vi "peis.vi"(5 "Draw":T2(ring), 6 "DLLPath":path, 7 "Channel":u8(ring) items=["1", "2", "3", "4", "5", "6", "7", "8", "9", "10", "11", "12", "13", "14", "15", "16"], 8 "error in (no error)":errorcluster, 9 "PEIS Parameters":T3={"Step_number"=0, "Initial_Voltage_step"=0.0, "vs_initial"=TRUE, "Final_Voltage_step"=1.0, "vs_final"=FALSE, "Duration_step"=1.0, "Record_every_dI"=0.1, "Record_every_dT"=0.1, "Initial_frequency"=100000.0, "sweep"=FALSE, "Final_frequency"=1.0, "Frequency_number"=51, "Amplitude_Voltage"=0.01, "Wait_for_steady"=2.0, "Average_N_times"=1, "Correction"=TRUE, "I_Range"=12, "Bandwidth"=5, "em"=1, "ce"=0} {"ce" items=["Standard", "CE to ground"]; "Initial_Voltage_step" min=-10 max=10 format="%.5f"; "Step_number" min=0 step=1; "I_Range" items=["1pA", "1nA", "10nA", "100nA", "1µA", "10µA", "100µA", "1mA", "10mA", "100mA", "1A", "Booster", "Auto"]; "Wait_for_steady" min=0 format="%.2f"; "Record_every_dT" min=0 format="%.2e"; "Record_every_dI" min=0 format="%.2e"; "Duration_step" min=0 format="%.5f"; "Final_Voltage_step" min=-10 max=10 format="%.5f"; "Bandwidth" items=["1"=1, "2"=2, "3"=3, "4"=4, "5"=5, "6"=6, "7"=7, "8"=8, "9"=9]; "Average_N_times" min=1 max=1000 step=1; "Amplitude_Voltage" min=0.0005 max=0.5 format="%.2e"; "Final_frequency" min=1e-05 max=1000000 format="%.2e"; "Frequency_number" min=1 max=10000; "Initial_frequency" min=1e-05 max=1000000 format="%.2e"}, 11 "IP adress":string="192.109.209.229") -> (0 "error out":errorcluster, 2 "Exit 2":bool=TRUE, 3 "XY Graph":cluster{"Data p1":sgl[], "Data p1":dbl[]}[](graph), 4 "Data":T1)   [LabVIEW 2022 SP3]
doc: "The Staircase Potentio Electrochemical Impedance Spectroscopy (SPEIS) technique is designed to perform successive impedance measurements (on a whole frequency range) during a potential sweep. \nThis technique consists in a staircase potential sweep (potential limits and number of steps defined by the user). An impedance measurement (with an adjustable number of frequencies) is performed on each potential step.\n\nIn general, in this VI, the first thing to do is to start by establishing the connection with the instrument defined by its IP adress, then load the firmware in the channel selected, get the information on the plugged channels, load protocol on a channel, start/stop the protocol, retreive data and draw the graph.\nThis technique is applied just for channels with impedance capabilities (Zboard)."
uses:
  Library/EClib Functions/PEISParameters.ctl
  Library/EClib Functions/Parameters.ctl
  Library/EClib Functions/EClib functions.lvlib
panel:
  in  "Display Parameters?":bool caption="Display Parameters"
  out "DllPath":path caption="DLL Path"
  out "LibVersion":string caption="DLL Version"
  out "Number of points":i32=52
  out "Data p0":sgl[][](array[numeric])=[[0.100008, 0.099745475, 1.9343544e-05], [0.200016, 0.09966919, 1.936642e-05], [0.300024, 0.10005063, 1.9374045e-05], [0.400032, 0.10005063, 1.9358795e-05], [0.50004, 0.09997434, 1.9358795e-05], [0.600048, 0.09982177, 1.938167e-05], [0.700056, 0.099516615, 1.9358795e-05], [0.800064, 0.099898055, 1.9374045e-05], [0.90007204, 0.099516615, 1.936642e-05]]
  out "Data p1":sgl[][](array[numeric])=[[99999.99, 0.009897927, 1.5485124e-05, -0.23932889, 0.09957624, 2.0601647e-05, 0.0, 0.017584162, 1.5528842e-05, -0.13801742, -0.10928005, -2.0601661e-05, 0.0, 1.89, 7.0], [79789.055, 0.009909321, 1.4999416e-05, -0.28277892, 0.09956935, 2.0610883e-05, 0.0, 0.017358849, 1.5026583e-05, -0.16497254, -0.10927754, -2.0610896e-05, 0.0, 2.319, 7.0], [63671.867, 0.00993305, 1.4371862e-05, -0.3338619, 0.099571265, 2.0617736e-05, 0.0, 0.01701651, 1.4388475e-05, -0.19887781, -0.10927467, -2.0617748e-05, 0.0, 2.748, 7.0], [50804.684, 0.009895762, 1.349999e-05, -0.38682938, 0.099595726, 2.0621628e-05, 0.0, 0.016509676, 1.3509973e-05, -0.23511207, -0.10929042, -2.0621641e-05, 0.0, 3.177, 7.0], [40539.06, 0.009924297, 1.2531375e-05, -0.43154812, 0.09956674, 2.0623062e-05, 0.0, 0.01605967, 1.2537333e-05, -0.27001935, -0.1092824, -2.0623074e-05, 0.0, 3.606, 7.0], [32343.752, 0.009929493, 1.1422184e-05, -0.4605673, 0.099575475, 2.0627644e-05, 0.0, 0.015497766, 1.1425662e-05, -0.29694676, -0.10927959, -2.0627656e-05, 0.0, 4.035, 7.0], [25812.496, 0.009931898, 1.0332502e-05, -0.47349262, 0.09957423, 2.0616248e-05, 0.0, 0.014982226, 1.0334525e-05, -0.31350675, -0.10928383, -2.0616259e-05, 0.0, 4.4639997, 7.0], [20593.748, 0.009683827, 9.104932e-06, -0.46709442, 0.09957324, 2.0613099e-05, 0.0, 0.014134236, 9.106069e-06, -0.3174526, -0.10928545, -2.0613114e-05, 0.0, 4.75, 7.0], [16429.69, 0.00984061, 8.381006e-06, -0.4425385, 0.0995779, 2.0614962e-05, 0.0, 0.013980997, 8.381673e-06, -0.30736777, -0.10928426, -2.0614974e-05, 0.0, 5.036, 7.0], [13109.373, 0.009880392, 7.759602e-06, -0.4042132, 0.09956233, 2.0629059e-05, 0.0, 0.013766184, 7.759997e-06, -0.28469434, -0.10927877, -2.0629072e-05, 0.0, 5.322, 7.0], [10460.936, 0.009915135, 7.290463e-06, -0.35881066, 0.099576354, 2.062228e-05, 0.0, 0.013552605, 7.2907023e-06, -0.25464892, -0.10927802, -2.0622294e-05, 0.0, 5.608, 7.0], [8351.5625, 0.009958473, 6.968417e-06, -0.30687237, 0.09957134, 2.0619169e-05, 0.0, 0.013452288, 6.968562e-06, -0.21966934, -0.10928822, -2.0619183e-05, 0.0, 5.894, 7.0], [6660.1553, 0.009773157, 6.585265e-06, -0.26302314, 0.09957721, 2.0628519e-05, 0.0, 0.013077308, 6.5853465e-06, -0.18975565, -0.109301746, -2.0628531e-05, 0.0, 6.0620003, 7.0], [5313.953, 0.009875495, 6.4977903e-06, -0.21722555, 0.09959636, 2.061105e-05, 0.0, 0.013129692, 6.497844e-06, -0.15612268, -0.10930546, -2.0611064e-05, 0.0, 6.269, 7.0], [4241.786, 0.009916322, 6.4091464e-06, -0.17841792, 0.09959986, 2.0643229e-05, 0.0, 0.013149473, 6.4091746e-06, -0.12683374, -0.109303646, -2.0643243e-05, 0.0, 6.4830003, 7.0], [3385.4163, 0.009962957, 6.371731e-06, -0.15283132, 0.09959816, 2.0641255e-05, 0.0, 0.013166811, 6.371748e-06, -0.11219756, -0.10930573, -2.0641268e-05, 0.0, 6.697, 7.0], [2699.3184, 0.009985389, 6.3324687e-06, -0.12883663, 0.099599674, 2.0642745e-05, 0.0, 0.013169419, 6.3324833e-06, -0.09362733, -0.10931173, -2.0642758e-05, 0.0, 6.9110003, 7.0], [2153.4448, 0.009996085, 6.3133293e-06, -0.11305499, 0.09959159, 2.0643656e-05, 0.0, 0.013185124, 6.313335e-06, -0.08275235, -0.109307505, -2.064367e-05, 0.0, 7.125, 7.0], [1717.748, 0.010014333, 6.2567524e-06, -0.10080016, 0.09959457, 2.0655203e-05, 0.0, 0.013182044, 6.256763e-06, -0.07431483, -0.10931141, -2.0655216e-05, 0.0, 7.34, 7.0], [1372.1951, 0.010016238, 6.2877625e-06, -0.09321749, 0.09959682, 2.064688e-05, 0.0, 0.013175669, 6.2877634e-06, -0.06877315, -0.10931128, -2.0646892e-05, 0.0, 7.5550003, 7.0], [1096.7545, 0.010012516, 6.286433e-06, -0.08541584, 0.09960139, 2.0640491e-05, 0.0, 0.013178928, 6.2864306e-06, -0.062073976, -0.10930484, -2.0640506e-05, 0.0, 7.77, 7.0], [871.93097, 0.010010969, 6.268487e-06, -0.08781743, 0.09959833, 2.0634905e-05, 0.0, 0.013172707, 6.2684835e-06, -0.06440747, -0.109307244, -2.0634918e-05, 0.0, 7.987, 7.0], [696.1138, 0.01003125, 6.2508416e-06, -0.093888, 0.09959319, 2.0650714e-05, 0.0, 0.013164024, 6.2508466e-06, -0.069969416, -0.10931639, -2.0650728e-05, 0.0, 8.203, 7.0], [555.8894, 0.010025321, 6.2520185e-06, -0.10746312, 0.099596396, 2.063822e-05, 0.0, 0.01315077, 6.2520166e-06, -0.08037281, -0.109306626, -2.0638234e-05, 0.0, 8.42, 7.0], [443.43906, 0.010033136, 6.209101e-06, -0.12175393, 0.0995993, 2.0631758e-05, 0.0, 0.01312816, 6.2091035e-06, -0.091670275, -0.109299496, -2.063177e-05, 0.0, 8.639, 7.0], [353.75473, 0.01003465, 6.1840165e-06, -0.14335668, 0.09959073, 2.0645593e-05, 0.0, 0.013097799, 6.1840187e-06, -0.10758209, -0.10931424, -2.0645608e-05, 0.0, 8.859, 7.0], [281.8943, 0.010030967, 6.109471e-06, -0.17281115, 0.09959446, 2.0650212e-05, 0.0, 0.013065848, 6.109473e-06, -0.129511, -0.10930905, -2.0650225e-05, 0.0, 9.0789995, 7.0], [225.3606, 0.010023677, 6.0119432e-06, -0.20512176, 0.09959748, 2.064375e-05, 0.0, 0.013001974, 6.0119396e-06, -0.15545309, -0.1093129, -2.0643763e-05, 0.0, 9.301, 7.0], [180.28844, 0.010028235, 5.913567e-06, -0.25207758, 0.0995884, 2.0643136e-05, 0.0, 0.012923154, 5.913563e-06, -0.19031943, -0.1093126, -2.0643149e-05, 0.0, 9.526, 7.0], [143.75787, 0.010025335, 5.723294e-06, -0.2980666, 0.09959362, 2.0638052e-05, 0.0, 0.012791262, 5.7232987e-06, -0.22673774, -0.109312676, -2.0638066e-05, 0.0, 9.755, 7.0], [114.59661, 0.0100282775, 5.478785e-06, -0.36026663, 0.09959826, 2.0642558e-05, 0.0, 0.012615283, 5.4787893e-06, -0.27884817, -0.109307505, -2.0642572e-05, 0.0, 9.987, 7.0], [91.552734, 0.010020258, 5.1631105e-06, -0.41180015, 0.09958356, 2.0632298e-05, 0.0, 0.012400166, 5.1631077e-06, -0.32256132, -0.10930771, -2.0632311e-05, 0.0, 10.219, 7.0], [72.87778, 0.010045694, 4.7920767e-06, -0.47027957, 0.0995903, 1.9318108e-05, 0.0, 0.012195916, 4.7920753e-06, -0.37585485, -0.10930665, -1.931812e-05, 0.0, 10.735, 6.0], [58.30223, 0.010017018, 4.3459513e-06, -0.5196618, 0.09958969, 1.931711e-05, 0.0, 0.011869716, 4.345951e-06, -0.41790736, -0.109305374, -1.9317124e-05, 0.0, 10.989, 6.0], [46.50297, 0.010043655, 3.8964367e-06, -0.5461425, 0.09958527, 1.9321726e-05, 0.0, 0.011661541, 3.8964395e-06, -0.45622373, -0.10929812, -1.9321737e-05, 0.0, 11.24, 6.0], [36.95101, 0.0100237075, 3.4589034e-06, -0.55786407, 0.09959118, 1.9322812e-05, 0.0, 0.011445447, 3.4589052e-06, -0.47548974, -0.1093029, -1.9322824e-05, 0.0, 11.498, 6.0], [29.592804, 0.010024518, 3.0782626e-06, -0.5442606, 0.099590674, 1.9320825e-05, 0.0, 0.011281099, 3.0782635e-06, -0.4723431, -0.10930497, -1.9320838e-05, 0.0, 11.782001, 6.0], [23.588463, 0.010025413, 2.7635026e-06, -0.50970626, 0.09959939, 1.931987e-05, 0.0, 0.011168829, 2.7635024e-06, -0.45203626, -0.10930516, -1.9319881e-05, 0.0, 12.092, 6.0], [18.780045, 0.010028319, 2.5114025e-06, -0.46162716, 0.0995976, 1.9318664e-05, 0.0, 0.01109292, 2.5114036e-06, -0.4128492, -0.109315775, -1.9318675e-05, 0.0, 12.425, 6.0], [15.024037, 0.010029642, 2.331001e-06, -0.4064955, 0.099582985, 1.9321948e-05, 0.0, 0.01104459, 2.3310024e-06, -0.36793888, -0.10930361, -1.9321958e-05, 0.0, 12.772, 6.0], [11.982363, 0.010013976, 2.1986236e-06, -0.3445742, 0.0995901, 1.9318428e-05, 0.0, 0.01101896, 2.198625e-06, -0.31417423, -0.10929007, -1.931844e-05, 0.0, 13.119, 6.0], [9.574144, 0.010021789, 2.1110484e-06, -0.29042864, 0.09959056, 1.931938e-05, 0.0, 0.011009957, 2.1110482e-06, -0.26570365, -0.10930588, -1.9319392e-05, 0.0, 13.55, 6.0], [7.6293964, 0.010015764, 2.047544e-06, -0.2358973, 0.09959619, 1.9324216e-05, 0.0, 0.010986972, 2.0475438e-06, -0.21676749, -0.10930043, -1.9324229e-05, 0.0, 14.088, 6.0], [6.084501, 0.010008753, 2.0095065e-06, -0.19609833, 0.09960107, 1.9321422e-05, 0.0, 0.010978085, 2.0095063e-06, -0.17923641, -0.10930903, -1.9321435e-05, 0.0, 14.758, 6.0], [4.858519, 0.0100127505, 1.9834858e-06, -0.15383446, 0.099605374, 1.9325236e-05, 0.0, 0.01099137, 1.983485e-06, -0.14275539, -0.10930968, -1.9325249e-05, 0.0, 15.594, 6.0], [3.8752477, 0.010018873, 1.964741e-06, -0.12660927, 0.09960577, 1.9319072e-05, 0.0, 0.01098087, 1.9647398e-06, -0.11773729, -0.10930894, -1.9319084e-05, 0.0, 16.639, 6.0], [3.1001983, 0.01002199, 1.954336e-06, -0.101673305, 0.09960291, 1.9318823e-05, 0.0, 0.010977447, 1.9543347e-06, -0.09406805, -0.10931086, -1.9318833e-05, 0.0, 17.943, 6.0], [2.4660668, 0.010017678, 1.9471984e-06, -0.08063111, 0.09960053, 1.9318097e-05, 0.0, 0.010982101, 1.9471975e-06, -0.07494378, -0.10931104, -1.9318108e-05, 0.0, 19.579, 6.0], [1.9649143, 0.01001538, 1.9460967e-06, -0.064157724, 0.09960199, 1.9316354e-05, 0.0, 0.010980325, 1.946096e-06, -0.06017399, -0.1093061, -1.9316365e-05, 0.0, 21.627, 6.0], [1.5725644, 0.010012327, 1.941652e-06, -0.051375534, 0.09960348, 1.9317453e-05, 0.0, 0.010977772, 1.9416514e-06, -0.04843211, -0.10930792, -1.9317464e-05, 0.0, 24.183, 6.0], [1.2520034, 0.010019626, 1.939335e-06, -0.041469768, 0.09961237, 1.9318904e-05, 0.0, 0.010981496, 1.9393347e-06, -0.038478374, -0.109313786, -1.9318915e-05, 0.0, 27.391, 6.0], [1.0016024, 0.010014649, 1.938777e-06, -0.033258826, 0.09960662, 1.931856e-05, 0.0, 0.010977961, 1.9387764e-06, -0.031450033, -0.109310396, -1.9318572e-05, 0.0, 31.398, 6.0]]
  in  "stop":bool
  in  "Exit":bool
  in  "Start":bool
  # "Instructions:\nBefore running the VI you must type a valid IP adress that corresponds to the instrument.Then press the Run button to execute this VI.\nWhile this VI is running, choose the available channel, enter the SPEIS parameters or keep the default\n values, then press the start button to begin the experience. \nChoose the waveform to draw : Nyquist, modZ, theta...\nPress the stop button to end experience and the exit button to stop the VI execution."
  # "Set E (V)  vs. previous"
  # "Before EIS  stay for ts (s)"
  # "and record every dI (A)"
  # "or every dt (s)"
  # "Start EIS from  Fi (Hz)"
  # "sweep linear/logarithmic"
  # "to Ff (Hz)"
  # "for Nf frequencies"
  # "with the amplitude (V)"
  # "wait for Pw"
  # "average Na times"
  # "drift correction"
  # "with I Range"
  # "and bandwidth"
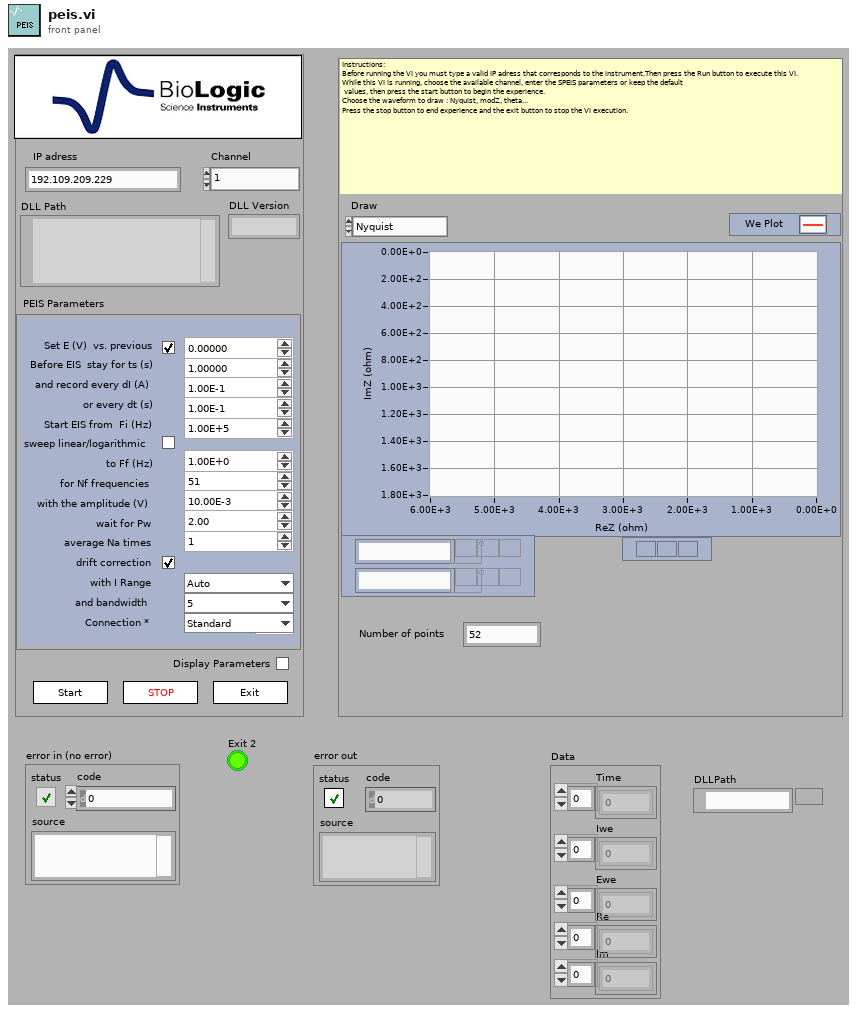
[diagram p1: front panel]
types:
  T1 = cluster{"Time":sgl[], "Iwe":sgl[], "Ewe":sgl[], "Re":sgl[], "Im":sgl[]}
  T2 = enum16{"Nyquist", "modZ", "theta", "modE", "modI", "Edc", "Idc", "E range", "I range", "f(t)", "Test"}
  T3 = typedef "EClib functions.lvlib/PEISParameters.ctl" = cluster{"Step_number":i32, "Initial_Voltage_step":sgl, "vs_initial":bool, "Final_Voltage_step":sgl, "vs_final":bool, "Duration_step":sgl, "Record_every_dI":sgl, "Record_every_dT":sgl, "Initial_frequency":sgl, "sweep":bool, "Final_frequency":sgl, "Frequency_number":i32, "Amplitude_Voltage":sgl, "Wait_for_steady":sgl, "Average_N_times":i32, "Correction":bool, "I_Range":u16, "Bandwidth":u16, "em":u16, "ce":u16}
  T4 = cluster{"LibVersion":string, "StringLength":u32, "DllPath":path}
  T5 = cluster{"Channel":i32, "BoardVersion":i32, "BoardSerialCode":i32, "FirmwareCode":i32, "FirmwareVersion":i32, "XilinxVersion":i32, "AmpCode":i32, "NbAmp":i32, "LcBoard":i32, "Zboard":i32, "MuxBoard":i32, "GPRAboard":i32, "MemSize":i32, "MemFilled":i32, "state":i32, "MaxIRange":i32, "MinIRange":i32, "MaxBandwidth":i32, "NbOfTechniques":i32}
  T6 = typedef "EClib functions.lvlib/Parameters.ctl" = enum16{"CA", "CASG", "CP", "GEIS", "ISCAN", "OCV", "PEIS", "SCCX", "SGEIS", "SPEIS", "VSCAN", "MP"}
  T7 = typedef "EClib functions.lvlib/TechniqueParameters.ctl" = cluster{"String Label":string, "Type":i32, "Valeur":i32, "Index":i32}
  T8 = cluster{"string before end tag":string, i32, i32, i32}[]
  T9 = cluster{"IRQskipped":i32, "NbRaws":i32, "NbCols":i32, "Technique Index":i32, "TechniqueID":i32, "PrcessIndex":i32, "loop":i32, "StartTime":dbl, "MuxPad":i32}
  T10 = cluster{"State":i32, "MemFilled":i32, "TimeBase":sgl, " Ewe":sgl, " EweRangeMin":sgl, " EweRangeMax":sgl, "Ece":sgl, "EceRangeMin":sgl, "EceRangeMax":sgl, "Eoverflow":i32, "I":sgl, "IRange":i32, "Ioverflow":i32, "ElapsedTime":sgl, "Freq":sgl, "Rcomp":sgl, "Saturation":sgl, "OptErr":i32, "OptPos":i32}
  T11 = cluster{"Data p0":sgl[], "Data p0":sgl[], "Data p0":sgl[], sgl[], sgl[]}
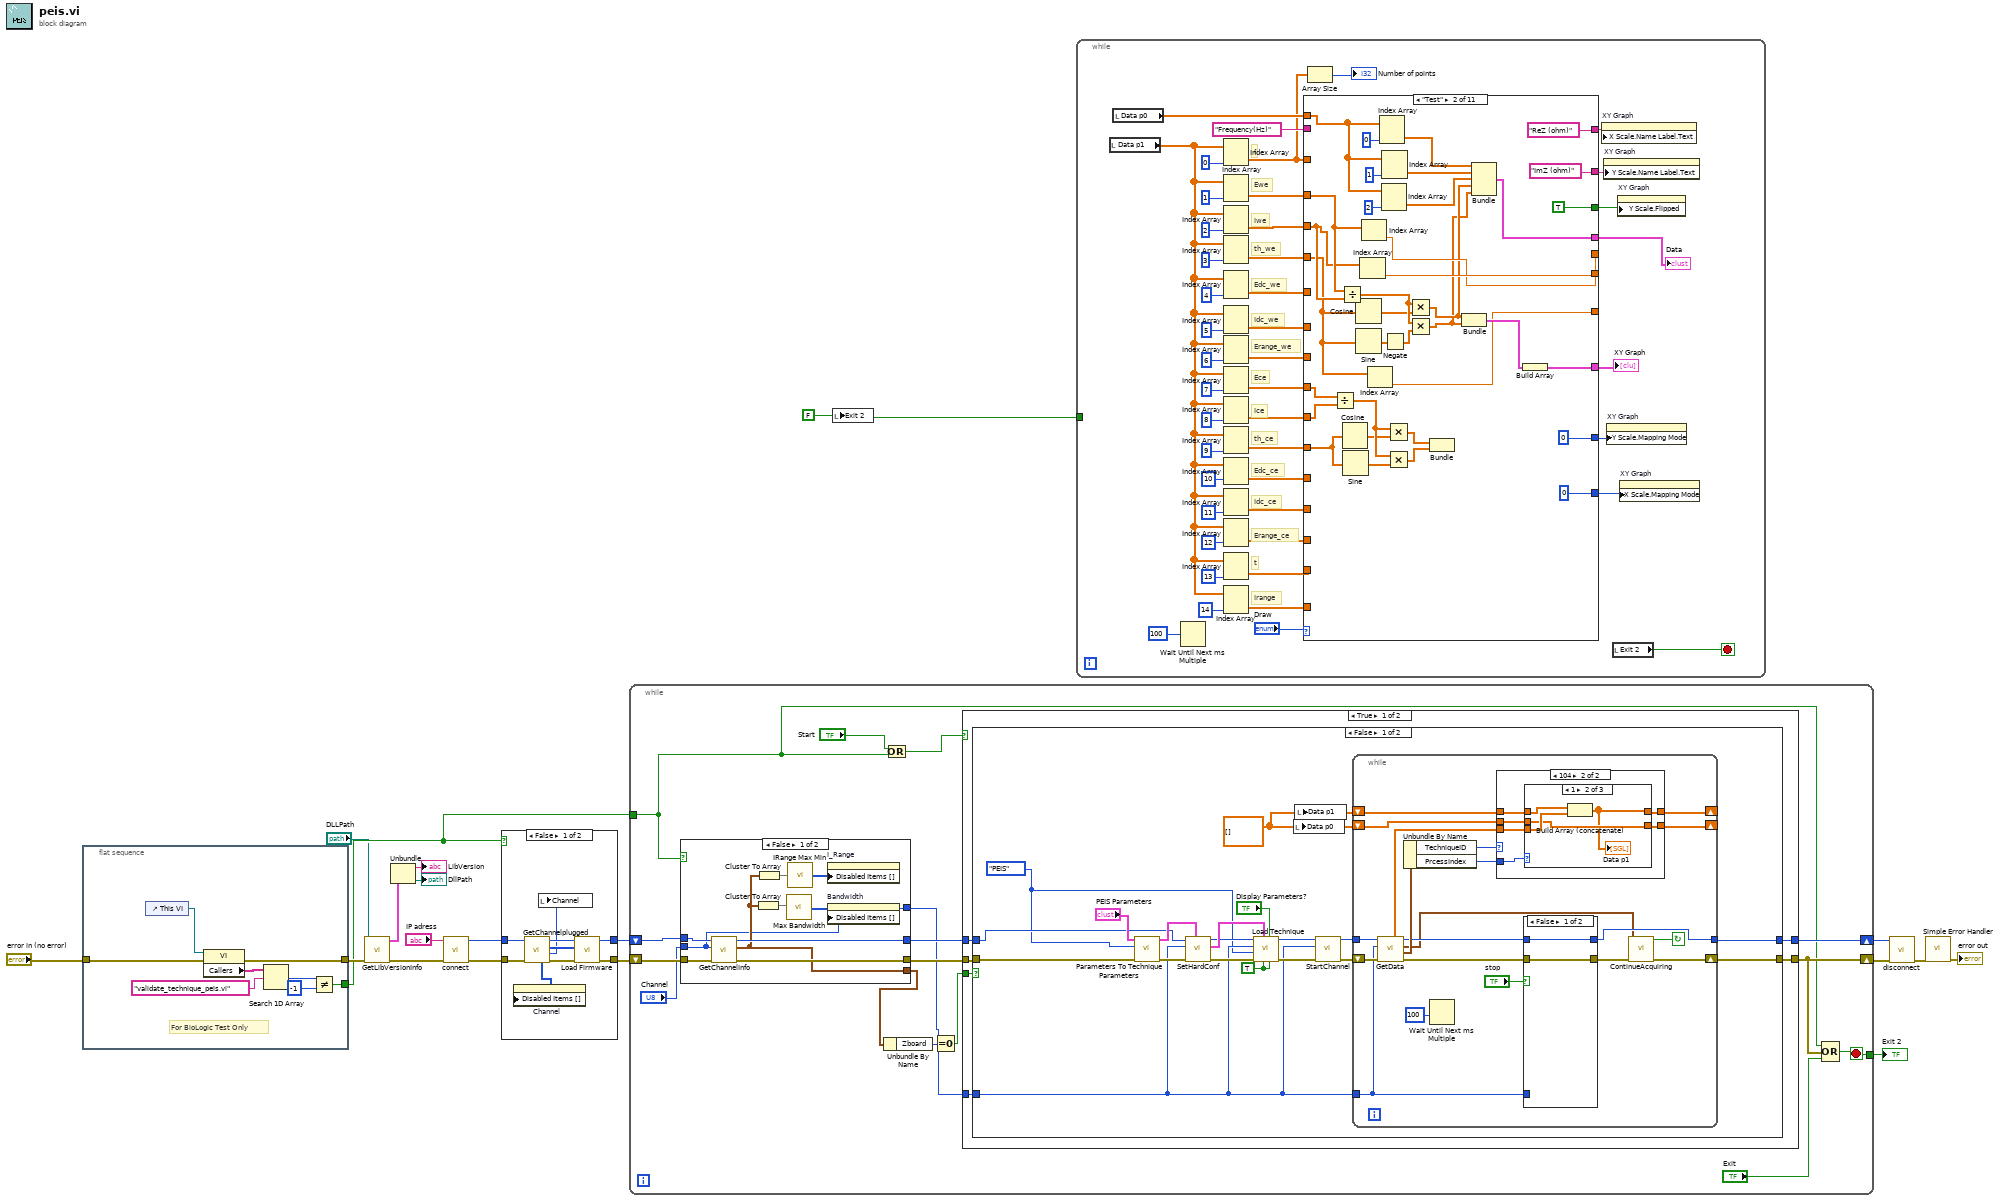
[diagram p0: block diagram]
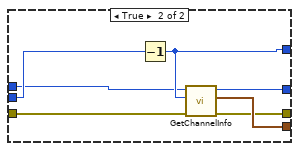
[diagram p3: hidden frame]
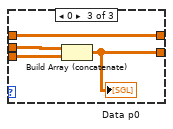
[diagram p6: hidden frame]
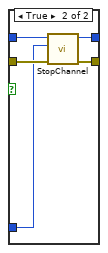
[diagram p7: hidden frame]
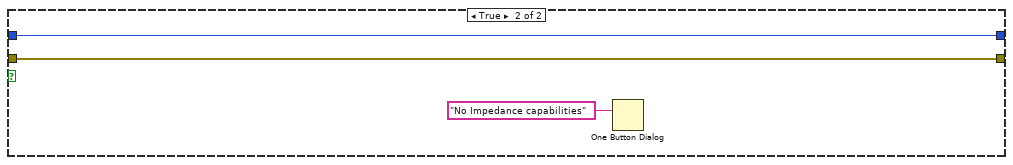
[diagram p8: hidden frame]
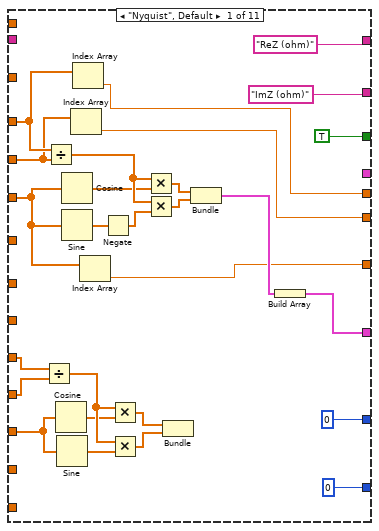
[diagram p10: hidden frame]
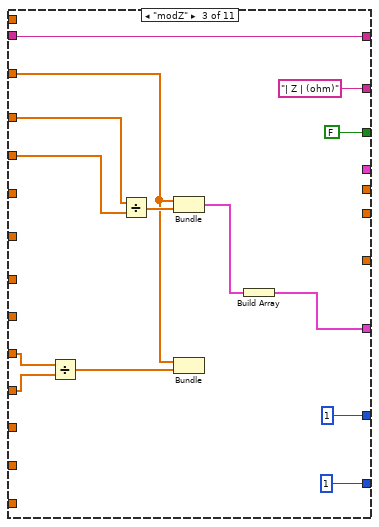
[diagram p11: hidden frame]
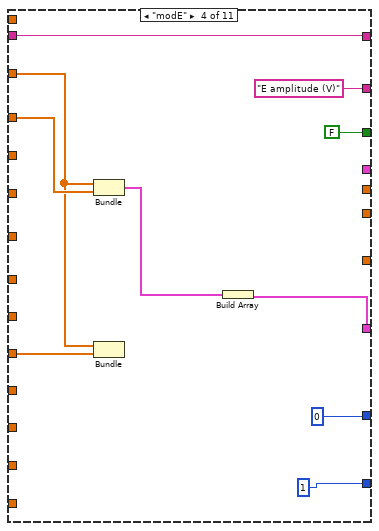
[diagram p12: hidden frame]
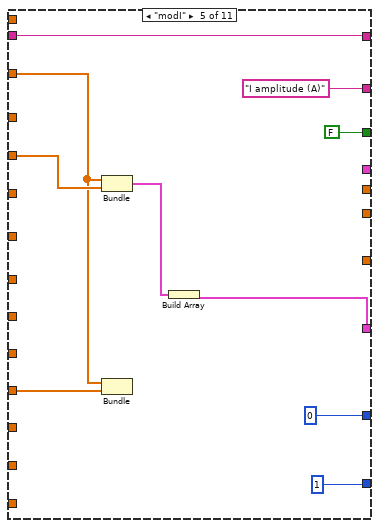
[diagram p13: hidden frame]
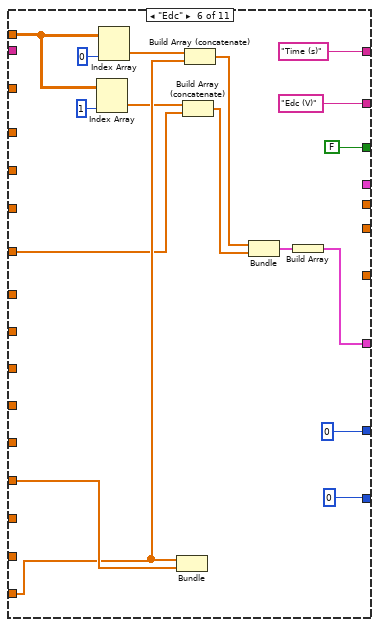
[diagram p14: hidden frame]
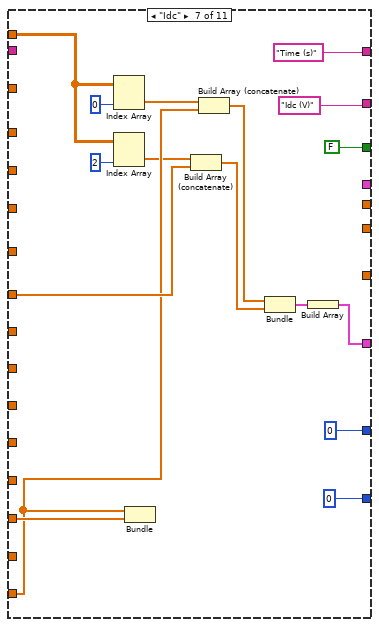
[diagram p15: hidden frame]
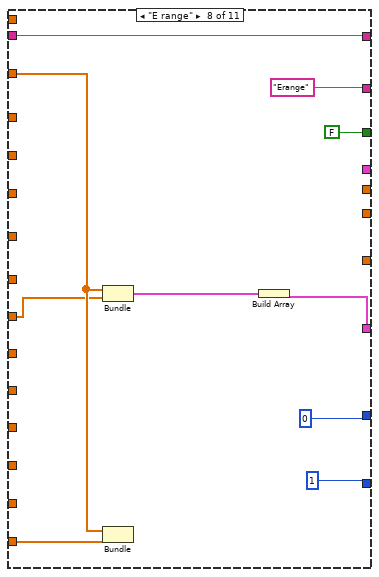
[diagram p16: hidden frame]
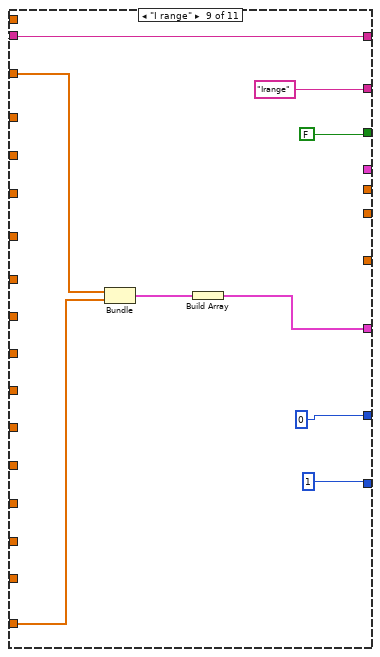
[diagram p17: hidden frame]
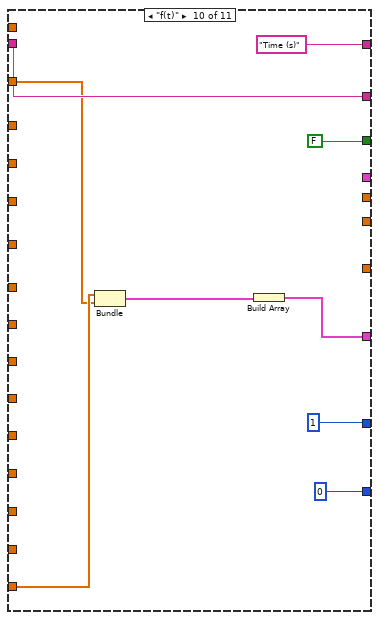
[diagram p18: hidden frame]
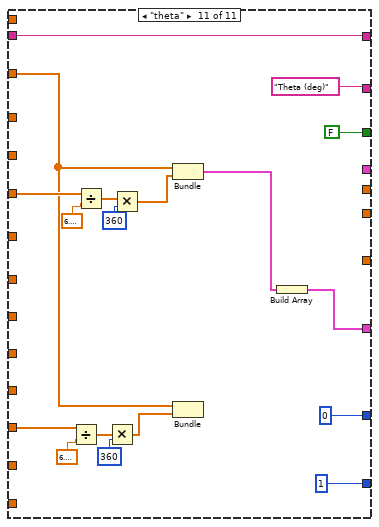
[diagram p19: hidden frame]
diagram:
  w18 = FALSE
  n1 = flat-sequence {
    tunnel: "error in (no error)" -> [w26]
    tunnel: [w25] -> w5
    tunnel: [w20] -> w3
    frame #0 {
      # "For BioLogic Test Only"
      n2 = control-ref of="This VI"() -> (w27:refnum<vi>)
      n3 = property class="VI"(reference=w27, error in=w26) -> (error out=w25:errorcluster, "Callers"=w24:string[])  [unwired: 1 out]
      n4 = Search 1D Array(1D array=w24, element="validate_technique_peis.vi") -> (index of element=w22:i32)  [unwired: 1 in]
      n5 = Not Equal?(x=w22, y=-1) -> (x != y?=w20:bool)
    }
  }
  n6 = call "GetLibVersionInfo.vi"("error in (no error)"=w5, "DLLPath"="DLLPath") -> ("error out"=w6:errorcluster, "LibInfo"=w9:T4)  [unwired: 8 in]
  n7 = Unbundle(w9) -> ("LibVersion"=→"LibVersion":string, "DllPath"=→"DllPath":path)  [unwired: 1 out]
  n8 = call "connect.vi"("error in (no error)"=w6, "IP"="IP adress") -> ("error out"=w15:errorcluster, "ID Out"=w17:i32)  [unwired: 5 in, 3 out]
  n9 = case shown="False" w3 {
    tunnel: w17 -> [w36 w38]
    tunnel: w15 -> [w35 w37]
    tunnel: [w30 w37] -> w14
    tunnel: [w29 w38] -> w13
    frame False {
      n10 = call "GetChannelplugged.vi"("error in (no error)"=w35, "ID In"=w36) -> ("error out"=w34:errorcluster, "FirstPluggedChannel"=w28:u8, "PluggedChannels"=w32:u8[], "ID Out"=w31:i32, "DisabledChannels"=w33:i32[])  [unwired: 5 in]
      n11 = property on="Channel" class="Ring (strict)"("Disabled Items []"=w33) -> ()  [unwired: 2 in, 2 out]
      n12 = local write "Channel"(w28) -> ()
      n13 = call "Load Firmware.vi"("error in (no error)"=w34, "Channels"=w32, "ID In"=w31) -> ("error out"=w30:errorcluster, "ID Out"=w29:i32)  [unwired: 6 in, 1 out]
    }
    frame True {
    }
  }
  n14 = while {
    shift-right: [w48] -> w12
    shift-left: w14 -> [w53]
    shift-right: [w54] -> w16
    shift-left: w13 -> [w52]
    tunnel: [w46] -> w10
    tunnel: w3 -> [w39]
    stop <- w46 stop-if-true
    n15 = case shown="False" w39 {
      tunnel: w53 -> [w64 w65]
      tunnel: w52 -> [w63 w66]
      tunnel: "Channel" -> [w55 w70]
      tunnel: [w62 w67] -> w50
      tunnel: [w61 w68] -> w49
      tunnel: [w60 w71] -> w44
      tunnel: [w55 w69] -> w42
      frame False {
        n16 = call "GetChannelInfo.vi"("error in (no error)"=w64, "Channel"=w55, "ID"=w63) -> ("error out"=w61:errorcluster, "Channel information"=w60:T5, "ID Out"=w62:i32)  [unwired: 6 in]
        n17 = Cluster To Array(cluster=w60) -> (array=w58:i32[])
        n18 = Cluster To Array(cluster=w60) -> (array=w59:i32[])
        n19 = call "Max Bandwidth.vi"("resources"=w58) -> ("disabled ranges"=w57:i32[])
        n20 = call "IRange Max Min.vi"("resources"=w59) -> ("disabled ranges"=w56:i32[])
        n21 = property on="I_Range" class="Ring (strict)"("Disabled Items []"=w56) -> ()  [unwired: 2 in, 2 out]
        n22 = property on="Bandwidth" class="Ring (strict)"("Disabled Items []"=w57) -> ()  [unwired: 2 in, 2 out]
      }
      frame True {
        n23 = Decrement(x=w70) -> (x-1=w69:u8)
        n24 = call "GetChannelInfo.vi"("error in (no error)"=w65, "Channel"=w69, "ID"=w66) -> ("error out"=w68:errorcluster, "Channel information"=w71:T5, "ID Out"=w67:i32)  [unwired: 6 in]
      }
    }
    n25 = Unbundle By Name(w44) -> ("Zboard"=w45:i32)
    n26 = Or(x="Start", y=w39) -> (x .or. y?=w40:bool)
    n27 = Equal To 0?(x=w45) -> (x = 0?=w43:bool)
    n28 = case shown="True" w40 {
      tunnel: w42 -> [w76 _]
      tunnel: [w77 w146] -> w48
      tunnel: w49 -> [w75 w146]
      tunnel: w43 -> [w74 _]
      tunnel: w50 -> [w73 w145]
      tunnel: [w72 w145] -> w54
      frame True {
        n29 = case shown="False" w74 {
          tunnel: [w96 w143] -> w77
          tunnel: w76 -> [w80 _]
          tunnel: w75 -> [w81 w143]
          tunnel: w73 -> [w79 w142]
          tunnel: [w89 w142] -> w72
          frame False {
            w78 = Parameters."PEIS" ("Parameters")
            w88 = TRUE ("First Protocol")
            w95 = sgl[][] [] ("Data")
            n30 = call "Parameters To Technique Parameters.vi"("error in (no error)"=w81, "Parameters"=w78, "ParameterIN"="PEIS Parameters") -> ("error out"=w87:errorcluster, "Params Values"=w83:T7[])  [unwired: 7 in]
            n31 = call "SetHardConf.vi"("Params Values"=w83, "error in (no error)"=w87, "Channel"=w80, "ID In"=w79) -> ("error out"=w86:errorcluster, "Params Values Trimed"=w85:T8, "ID Out"=w84:i32)  [unwired: 5 in]
            n32 = call "Load Technique.vi"("Last Protocol"=w88, "Display Parameters?"="Display Parameters?", "First Protocol"=w88, "TechniqueParameters"=w85, "error in (no error)"=w86, "Parameters"=w78, "Selected Channel"=w80, "ID In"=w84) -> ("error out"=w92:errorcluster, "ID  Out"=w91:i32)  [unwired: 1 in, 1 out]
            n33 = local write "Data p0"(w95) -> ()
            n34 = local write "Data p1"(w95) -> ()
            n35 = call "StartChannel.vi"("error in (no error)"=w92, "Channel"=w80, "ID In"=w91) -> ("error out"=w93:errorcluster, "ID Out"=w90:i32)  [unwired: 7 in]
            n36 = while {
              shift-right: [w103] -> w96
              shift-left: w93 -> [w116]
              shift-right: [w111] -> _
              shift-left: w95 -> [w112]
              shift-right: [w110] -> _
              shift-left: w95 -> [w109]
              tunnel: w80 -> [w97]
              tunnel: w90 -> [w106]
              tunnel: [w104] -> w89
              stop <- w113 continue-if-true
              n37 = call "GetData.vi"("error in (no error)"=w116, "Channel"=w97, "ID In"=w106) -> ("error out"=w114:errorcluster, "Data information"=w107:T9, "Current values"=w99:T10, "ID Out"=w105:i32, "Data"=w100:dbl[][])  [unwired: 1 in, 3 out]
              n38 = Unbundle By Name(w107) -> ("TechniqueID"=w101:i32, "PrcessIndex"=w98:i32)
              n39 = Wait Until Next ms Multiple(millisecond multiple=u32 100) -> ()  [unwired: 1 out]
              n40 = case shown="104" w101 {
                tunnel: w100 -> [_ w124]
                tunnel: w112 -> [w118 w123]
                tunnel: [w118 w122] -> w111
                tunnel: [w117 w121] -> w110
                tunnel: w109 -> [w117 w120]
                tunnel: w98 -> [_ w119]
                frame Default {
                }
                frame 104 {
                  n41 = case shown="1" w119 {
                    tunnel: w124 -> [_ w130 w134]
                    tunnel: w123 -> [w126 w129 w132]
                    tunnel: [w126 w127 w132] -> w122
                    tunnel: [w125 w128 w131] -> w121
                    tunnel: w120 -> [w125 w128 w133]
                    frame Default {
                    }
                    frame 1 {
                      n42 = Build Array (concatenate)(w129, w130) -> (w127:dbl[][])
                      "Data p1" <- w127
                    }
                    frame 0 {
                      n43 = Build Array (concatenate)(w133, w134) -> (w131:dbl[][])
                      "Data p0" <- w131
                    }
                  }
                }
              }
              n44 = case shown="False" "stop" {
                tunnel: [w136 w141] -> w102
                tunnel: w114 -> [w136 w140]
                tunnel: w105 -> [w135 w139]
                tunnel: [w135 w138] -> w104
                tunnel: w97 -> [_ w137]
                frame False {
                }
                frame True {
                  n45 = call "StopChannel.vi"("error in (no error)"=w140, "Channel"=w137, "ID In"=w139) -> ("error out"=w141:errorcluster, "ID Out"=w138:i32)  [unwired: 7 in]
                }
              }
              n46 = call "ContinueAcquiring.vi"("error in"=w102, "Current values"=w99) -> ("error out"=w103:errorcluster, "ContinueAcquiring?"=w113:bool)  [unwired: 8 in]
            }
          }
          frame True {
            n47 = One Button Dialog(message="No Impedance capabilities" ("error source (\" \")")) -> ()  [unwired: 1 in, 1 out]
          }
        }
      }
      frame False {
      }
    }
    n48 = Compound Arithmetic op=OR(w39, w48, "Exit") -> (w46:bool)
  }
  "Exit 2" <- w10
  n49 = local write "Exit 2"(w18) -> ()
  n50 = while {
    tunnel: w18 -> [_]
    stop <- w179 stop-if-true
    # "Erange_ce"
    # "Idc_ce"
    # "Edc_ce"
    # "th_ce"
    # "Ice"
    # "Ece"
    # "t"
    # "Irange"
    # "Erange_we"
    # "Idc_we"
    # "Edc_we"
    # "th_we"
    # "Iwe"
    # "Ewe"
    # "f"
    n51 = local read "Data p1"() -> (w164:sgl[][])
    n52 = local read "Data p0"() -> (w151:sgl[][])
    n53 = Wait Until Next ms Multiple(millisecond multiple=u32 100) -> ()  [unwired: 1 out]
    n54 = Index Array(array=w164, index (col)=0 ("Index")) -> (element=w150:sgl[])  [unwired: 1 in]
    n55 = Index Array(array=w164, index (col)=1 ("Index")) -> (element=w165:sgl[])  [unwired: 1 in]
    n56 = Index Array(array=w164, index (col)=2 ("Index")) -> (element=w169:sgl[])  [unwired: 1 in]
    n57 = Index Array(array=w164, index (col)=3 ("Index")) -> (element=w184:sgl[])  [unwired: 1 in]
    n58 = Index Array(array=w164, index (col)=4 ("disabled index (col)")) -> (element=w178:sgl[])  [unwired: 1 in]
    n59 = Index Array(array=w164, index (col)=5 ("disabled index (col)")) -> (element=w175:sgl[])  [unwired: 1 in]
    n60 = Index Array(array=w164, index (col)=6 ("index (row)")) -> (element=w166:sgl[])  [unwired: 1 in]
    n61 = Index Array(array=w164, index (col)=7) -> (element=w157:sgl[])  [unwired: 1 in]
    n62 = Index Array(array=w164, index (col)=8) -> (element=w156:sgl[])  [unwired: 1 in]
    n63 = Index Array(array=w164, index (col)=9) -> (element=w155:sgl[])  [unwired: 1 in]
    n64 = Index Array(array=w164, index (col)=10) -> (element=w154:sgl[])  [unwired: 1 in]
    n65 = Index Array(array=w164, index (col)=11) -> (element=w153:sgl[])  [unwired: 1 in]
    n66 = Index Array(array=w164, index (col)=12) -> (element=w152:sgl[])  [unwired: 1 in]
    n67 = Index Array(array=w164, index (col)=13 ("disabled index (col)")) -> (element=w167:sgl[])  [unwired: 1 in]
    n68 = Index Array(array=w164, index (col)=14 ("disabled index (col)")) -> (element=w168:sgl[])  [unwired: 1 in]
    n69 = case shown="\"Test\"" "Draw" {
      tunnel: w150 -> [_ _ w255 w269 w280 _ _ w325 w333 w342 w351]
      tunnel: w165 -> [w196 w234 w266 w276 _ _ _ _ _ _ _]
      tunnel: w169 -> [w195 w233 w259 _ w286 _ _ _ _ _ _]
      tunnel: ["ImZ (ohm)" ("Y Scale.Name Label.Text") "ImZ (ohm)" ("Y Scale.Name Label.Text") "| Z | (ohm)" ("Y Scale.Name Label.Text") "E amplitude (V)" ("Y Scale.Name Label.Text") "I amplitude (A)" ("Y Scale.Name Label.Text") "Edc (V)" ("Y Scale.Name Label.Text") "Idc (V)" ("Y Scale.Name Label.Text") "Erange" ("Y Scale.Name Label.Text") "Irange" ("Y Scale.Name Label.Text") w347 "Theta (deg)" ("Y Scale.Name Label.Text")] -> w186
      tunnel: w184 -> [w197 w221 _ _ _ _ _ _ _ _ w360]
      tunnel: ["ReZ (ohm)" ("Y Scale.Name Label.Text") "ReZ (ohm)" ("Y Scale.Name Label.Text") w263 w274 w284 "Time (s)" ("Y Scale.Name Label.Text") "Time (s)" ("Y Scale.Name Label.Text") w330 w339 "Time (s)" ("Y Scale.Name Label.Text") w366] -> w183
      tunnel: "Frequency(Hz)" ("Y Scale.Name Label.Text") -> [_ _ w263 w274 w284 _ _ w330 w339 w347 w366]
      tunnel: [TRUE ("Y Scale.Flipped") TRUE ("Y Scale.Flipped") FALSE ("Y Scale.Flipped") FALSE ("Y Scale.Flipped") FALSE ("Y Scale.Flipped") FALSE ("Y Scale.Flipped") FALSE ("Y Scale.Flipped") FALSE ("Y Scale.Flipped") FALSE FALSE FALSE ("Y Scale.Flipped")] -> w181
      tunnel: [u8 0 ("X Scale.Mapping Mode") u8 0 ("X Scale.Mapping Mode") u8 1 ("X Scale.Mapping Mode") u8 1 ("X Scale.Mapping Mode") u8 1 ("X Scale.Mapping Mode") 0 0 1 1 0 u8 1 ("X Scale.Mapping Mode")] -> w180
      tunnel: w178 -> [_ _ _ _ _ w287 _ _ _ _ _]
      tunnel: w175 -> [_ _ _ _ _ _ w308 _ _ _ _]
      tunnel: w166 -> [_ _ _ _ _ _ _ w321 _ _ _]
      tunnel: w168 -> [_ _ _ _ _ _ _ _ w334 _ _]
      tunnel: w167 -> [_ _ _ _ _ w289 w307 _ _ w343 _]
      tunnel: [0 0 1 u8 0 ("X Scale.Mapping Mode") u8 0 ("X Scale.Mapping Mode") 0 0 0 0 1 0 ("X Scale.Mapping Mode")] -> w171
      tunnel: w157 -> [w209 w244 w257 w270 _ _ _ _ _ _ _]
      tunnel: w156 -> [w208 w243 w256 _ w279 _ _ _ _ _ _]
      tunnel: w155 -> [w207 w242 _ _ _ _ _ _ _ _ w352]
      tunnel: w154 -> [_ _ _ _ _ w299 _ _ _ _ _]
      tunnel: w153 -> [_ _ _ _ _ _ w316 _ _ _ _]
      tunnel: w152 -> [_ _ _ _ _ _ _ w322 _ _ _]
      tunnel: [w202 w237 w253 w267 w277 w298 w314 w323 w331 w340 w349] -> w148
      tunnel: w151 -> [_ w226 _ _ _ w292 w310 _ _ _ _]
      tunnel: [w194 w232 _ _ _ _ _ _ _ _ _] -> _
      tunnel: [w193 w231 _ _ _ _ _ _ _ _ _] -> _
      tunnel: [w192 w230 _ _ _ _ _ _ _ _ _] -> _
      tunnel: [_ w222 _ _ _ _ _ _ _ _ _] -> w147
      frame "Nyquist", Default {
        n70 = Divide(x=w209, y=w208) -> (x/y=w204:sgl[])
        n71 = Divide(x=w196, y=w195) -> (x/y=w205:sgl[])
        n72 = Cosine(x=w207) -> (cos(x)=w203:sgl[])
        n73 = Sine(x=w207) -> (sin(x)=w210:sgl[])
        n74 = Cosine(x=w197) -> (cos(x)=w198:sgl[])
        n75 = Sine(x=w197) -> (sin(x)=w201:sgl[])
        n76 = Index Array(array=w195) -> (element=w194:sgl)  [unwired: 1 in]
        n77 = Index Array(array=w196) -> (element=w193:sgl)  [unwired: 1 in]
        n78 = Index Array(array=w197) -> (element=w192:sgl)  [unwired: 1 in]
        n79 = Negate(x=w201) -> (-x=w191:sgl[])
        n80 = Multiply(x=w204, y=w203) -> (x*y=w212:sgl[])
        n81 = Multiply(x=w204, y=w210) -> (x*y=w211:sgl[])
        n82 = Multiply(x=w205, y=w198) -> (x*y=w200:sgl[])
        n83 = Multiply(x=w205, y=w191) -> (x*y=w199:sgl[])
        n84 = Bundle(w212, w211) -> ()  [unwired: 1 in, 1 out]
        n85 = Bundle(w200, w199) -> (w206:cluster{sgl[], sgl[]})  [unwired: 1 in]
        n86 = Build Array(w206) -> (w202:cluster{sgl[], sgl[]}[])
      }
      frame "Test" {
        n87 = Divide(x=w244, y=w243) -> (x/y=w239:sgl[])
        n88 = Divide(x=w234, y=w233) -> (x/y=w240:sgl[])
        n89 = Cosine(x=w242) -> (cos(x)=w238:sgl[])
        n90 = Sine(x=w242) -> (sin(x)=w245:sgl[])
        n91 = Cosine(x=w221) -> (cos(x)=w235:sgl[])
        n92 = Sine(x=w221) -> (sin(x)=w236:sgl[])
        n93 = Index Array(array=w233) -> (element=w232:sgl)  [unwired: 1 in]
        n94 = Index Array(array=w234) -> (element=w231:sgl)  [unwired: 1 in]
        n95 = Index Array(array=w221) -> (element=w230:sgl)  [unwired: 1 in]
        n96 = Index Array(array=w226, index (col)=0 ("Index")) -> (element=w225:sgl[])  [unwired: 1 in]
        n97 = Index Array(array=w226, index (col)=2 ("Index")) -> (element=w223:sgl[])  [unwired: 1 in]
        n98 = Index Array(array=w226, index (col)=1 ("Index")) -> (element=w224:sgl[])  [unwired: 1 in]
        n99 = Negate(x=w236) -> (-x=w220:sgl[])
        n100 = Multiply(x=w239, y=w238) -> (x*y=w247:sgl[])
        n101 = Multiply(x=w239, y=w245) -> (x*y=w246:sgl[])
        n102 = Multiply(x=w240, y=w235) -> (x*y=w219:sgl[])
        n103 = Multiply(x=w240, y=w220) -> (x*y=w218:sgl[])
        n104 = Bundle(w247, w246) -> ()  [unwired: 1 in, 1 out]
        n105 = Bundle(w219, w218) -> (w241:cluster{sgl[], sgl[]})  [unwired: 1 in]
        n106 = Bundle("Data p0"=w225, "Data p0"=w224, "Data p0"=w223, w219, w218) -> (w222:T11)  [unwired: 1 in]
        n107 = Build Array(w241) -> (w237:cluster{sgl[], sgl[]}[])
      }
      frame "modZ" {
        n108 = Divide(x=w257, y=w256) -> (x/y=w258:sgl[])
        n109 = Divide(x=w266, y=w259) -> (x/y=w265:sgl[])
        n110 = Bundle("Data p1"=w255, w265) -> (w254:cluster{"Data p1":sgl[], sgl[]})  [unwired: 1 in]
        n111 = Bundle("Data p1"=w255, w258) -> ()  [unwired: 1 in, 1 out]
        n112 = Build Array(w254) -> (w253:cluster{"Data p1":sgl[], sgl[]}[])
      }
      frame "modE" {
        n113 = Bundle("Data p1"=w269, "Data p1"=w276) -> (w268:cluster{"Data p1":sgl[], "Data p1":sgl[]})  [unwired: 1 in]
        n114 = Bundle("Data p1"=w269, "Data p1"=w270) -> ()  [unwired: 1 in, 1 out]
        n115 = Build Array(w268) -> (w267:cluster{"Data p1":sgl[], "Data p1":sgl[]}[])
      }
      frame "modI" {
        n116 = Bundle("Data p1"=w280, "Data p1"=w286) -> (w278:cluster{"Data p1":sgl[], "Data p1":sgl[]})  [unwired: 1 in]
        n117 = Bundle("Data p1"=w280, "Data p1"=w279) -> ()  [unwired: 1 in, 1 out]
        n118 = Build Array(w278) -> (w277:cluster{"Data p1":sgl[], "Data p1":sgl[]}[])
      }
      frame "Edc" {
        n119 = Index Array(array=w292, index (col)=1 ("Index")) -> (element=w288:sgl[])  [unwired: 1 in]
        n120 = Index Array(array=w292, index (col)=0 ("Index")) -> (element=w290:sgl[])  [unwired: 1 in]
        n121 = Bundle("Data p1"=w289, "Data p1"=w299) -> ()  [unwired: 1 in, 1 out]
        n122 = Build Array (concatenate)(w288, w287) -> (w294:sgl[])
        n123 = Build Array (concatenate)(w290, w289) -> (w295:sgl[])
        n124 = Bundle(w295, w294) -> (w291:cluster{sgl[], sgl[]})  [unwired: 1 in]
        n125 = Build Array(w291) -> (w298:cluster{sgl[], sgl[]}[])
      }
      frame "Idc" {
        n126 = Index Array(array=w310, index (col)=0 ("Index")) -> (element=w309:sgl[])  [unwired: 1 in]
        n127 = Index Array(array=w310, index (col)=2 ("Index")) -> (element=w306:sgl[])  [unwired: 1 in]
        n128 = Bundle("Data p1"=w307, "Data p1"=w316) -> ()  [unwired: 1 in, 1 out]
        n129 = Build Array (concatenate)(w306, w308) -> (w304:sgl[])
        n130 = Build Array (concatenate)(w309, w307) -> (w305:sgl[])
        n131 = Bundle(w305, w304) -> (w315:cluster{sgl[], sgl[]})  [unwired: 1 in]
        n132 = Build Array(w315) -> (w314:cluster{sgl[], sgl[]}[])
      }
      frame "E range" {
        n133 = Bundle("Data p1"=w325, "Data p1"=w321) -> (w324:cluster{"Data p1":sgl[], "Data p1":sgl[]})  [unwired: 1 in]
        n134 = Bundle("Data p1"=w325, "Data p1"=w322) -> ()  [unwired: 1 in, 1 out]
        n135 = Build Array(w324) -> (w323:cluster{"Data p1":sgl[], "Data p1":sgl[]}[])
      }
      frame "I range" {
        n136 = Bundle("Data p1"=w333, "Data p1"=w334) -> (w332:cluster{"Data p1":sgl[], "Data p1":sgl[]})  [unwired: 1 in]
        n137 = Build Array(w332) -> (w331:cluster{"Data p1":sgl[], "Data p1":sgl[]}[])
      }
      frame "f(t)" {
        n138 = Bundle("Data p1"=w343, "Data p1"=w342) -> (w341:cluster{"Data p1":sgl[], "Data p1":sgl[]})  [unwired: 1 in]
        n139 = Build Array(w341) -> (w340:cluster{"Data p1":sgl[], "Data p1":sgl[]}[])
      }
      frame "theta" {
        n140 = Divide(x=w352, y=6.283185307179586) -> (x/y=w354:dbl[])
        n141 = Divide(x=w360, y=6.283185307179586) -> (x/y=w363:dbl[])
        n142 = Multiply(x=w354, y=360) -> (x*y=w356:dbl[])
        n143 = Multiply(x=w363, y=360) -> (x*y=w359:dbl[])
        n144 = Bundle("Data p1"=w351, w359) -> (w350:cluster{"Data p1":sgl[], dbl[]})  [unwired: 1 in]
        n145 = Bundle("Data p1"=w351, w356) -> ()  [unwired: 1 in, 1 out]
        n146 = Build Array(w350) -> (w349:cluster{"Data p1":sgl[], dbl[]}[])
      }
    }
    "XY Graph" <- w148
    "Data" <- w147
    n147 = Array Size(array=w150) -> (size(s)=→"Number of points":i32)
    n148 = property on="XY Graph" class="XYGraph (strict)"("X Scale.Name Label.Text"=w183) -> ()  [unwired: 2 in, 2 out]
    n149 = property on="XY Graph" class="XYGraph (strict)"("Y Scale.Name Label.Text"=w186) -> ()  [unwired: 2 in, 2 out]
    n150 = property on="XY Graph" class="XYGraph (strict)"("Y Scale.Mapping Mode"=w171) -> ()  [unwired: 2 in, 2 out]
    n151 = local read "Exit 2"() -> (w179:bool)
    n152 = property on="XY Graph" class="XYGraph (strict)"("Y Scale.Flipped"=w181) -> ()  [unwired: 2 in, 2 out]
    n153 = property on="XY Graph" class="XYGraph (strict)"("X Scale.Mapping Mode"=w180) -> ()  [unwired: 2 in, 2 out]
  }
  n154 = call "disconnect.vi"("error in (no error)"=w12, "ID In"=w16) -> ("error out"=w11:errorcluster)  [unwired: 9 in]
  n155 = call <vilib>:"Simple Error Handler.vi"("error in (no error)"=w11) -> ("error out"=→"error out":errorcluster)  [unwired: 4 in, 4 out]
